vi "MakeZlut.vi"   [LabVIEW 2011]
types:
  T1 = enum16{"init", "get", "set single frame", "set all"}
  T2 = cluster{"ROI1":i32, "Rmax (pix)":i32, "RminZ (pix)":i32, "LUTs":dbl[][][], "use trace":bool, "angular pixel\n coverage factor":dbl, "radial pixel\n coverage factor":dbl}
  T3 = typedef "IMAQ Image.ctl" = refnum<image>
  T4 = cluster{"front panel settings":cluster{"files":cluster{"LUT path":path, "Trace path":path, " folders #":i32, "base path":path, "use trace":bool, "use base":bool, "LUT tmp":i32, "Trace tmp":i32, "active path":path}, "Tracking":cluster{"RminZ (pix)":i32, "Rmax (pix)":i32, "angular pixel \ncoverage factor":dbl, "radial pixel \ncoverage factor":dbl}, "Frames":cluster{"Start frame":i32, "number of frames":u32, "display frame ":i32, "track every nd frame ":i32, "Track all frames":bool, "active frame":i32}, "Calibs":cluster{"Zlut number of steps":i32, "pix/um":dbl, "Z correction factor":dbl, "Zlut step size (um)":dbl, "ROI(pix)":i32}, "Beads":cluster{"number of ref beads":i32, "overlay":bool}, "Misc":cluster{"save images to new location":bool, "destination":path}}, "data":cluster{"Image":T3, "image size":i32[], "Bead Array":i32[][], "overlay image":T3, "# beads":i32, "Job list":string[][], "job running":bool, "job #":i32, "folders to go":i32}}
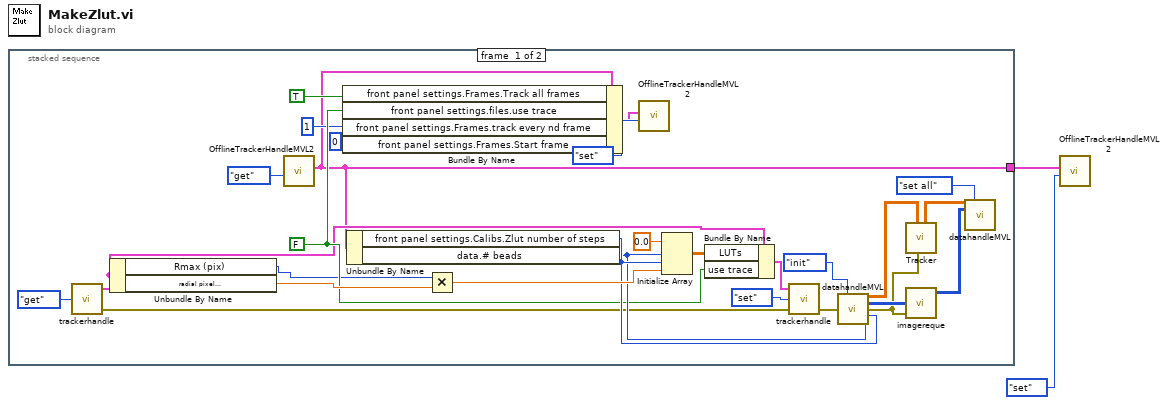
[diagram p0: block diagram]
diagram:
  n1 = stacked-sequence {
    tunnel: [w5 _] -> w1
    frame #0 {
      w9 = FALSE ("use trace")
      n2 = call "trackerhandle.vi"("action"=enum16{"get", "set"}."get") -> ("error out"=w7:errorcluster, "output Cluster"=w8:T2)  [unwired: 2 in, 1 out]
      n3 = Unbundle By Name(w8) -> ("Rmax (pix)"=w4:i32, "radial pixel\n coverage factor"=w16:dbl)
      n4 = call "OfflineTrackerHandleMVL2.vi"("action"=enum16{"get", "set"}."get") -> ("out"=w5:T4)  [unwired: 5 in, 1 out]
      n5 = Bundle By Name(cluster=w5, "front panel settings.Frames.Track all frames"=TRUE ("Track all frames"), "front panel settings.files.use trace"=w9, "front panel settings.Frames.track every nd frame"=1, "front panel settings.Frames.Start frame"=0) -> (w11:T4)
      n6 = Unbundle By Name(w5) -> ("front panel settings.Calibs.Zlut number of steps"=w14:i32, "data.# beads"=w13:i32)
      n7 = Multiply(x=w4, y=w16) -> (x*y=w17:dbl)
      n8 = call "OfflineTrackerHandleMVL2.vi"("action"=enum16{"get", "set"}."set", "in"=w11) -> ()  [unwired: 4 in, 2 out]
      n9 = Initialize Array(0.0 ("element"), w13, w14, w17) -> (w24:dbl[][][])
      n10 = Bundle By Name(cluster=w8, "LUTs"=w24, "use trace"=w9) -> (w26:T2)
      n11 = call "trackerhandle.vi"("error in"=w7, "action"=enum16{"get", "set"}."set", "input Cluster"=w26) -> ("error out"=w22:errorcluster)  [unwired: 2 out]
      n12 = call "datahandleMVL.vi"("action"=T1."init", "error in"=w22, "number of frames"=w14, "number of beads"=w13) -> ("XYZ out"=w30:dbl[][][], "time out"=w29:i32[][], "error in 2"=w18:errorcluster)  [unwired: 6 in, 3 out]
      n13 = call "Tracker.vi"("error in"=w18, "XYZdata in"=w30) -> ("XYZdata out"=w20:dbl[][][])  [unwired: 2 in, 7 out]
      n14 = call "imagereque.vi"("error in"=w18, "Time data in"=w29) -> ("Time data out"=w19:i32[][])  [unwired: 1 in, 2 out]
      n15 = call "datahandleMVL.vi"("xyz array in"=w20, "action"=T1."set all", "Time array in"=w19) -> ()  [unwired: 7 in, 6 out]
    }
    frame #1 {
    }
  }
  n16 = call "OfflineTrackerHandleMVL2.vi"("action"=enum16{"get", "set"}."set", "in"=w1) -> ()  [unwired: 4 in, 2 out]
